vi "TwoBallAuton3-12-14.vi"() -> ()   [LabVIEW 2014]
uses:
  TwoBallAuton.ctl
  Events.vi
  AutonVars.vi
panel:
  out "TargetDistance (In) ToReload":dbl=132.0
  out "Time Target (s)":dbl=3.0
  out "Y-Axis (Backward Speed)":dbl
  out "TargetDistance (In) ToFire":dbl=72.0
  out "Finish?":bool
  out "State":T1=enum."GetBall"
  # "Variables"
  # "Outputs"
  # "Inputs"
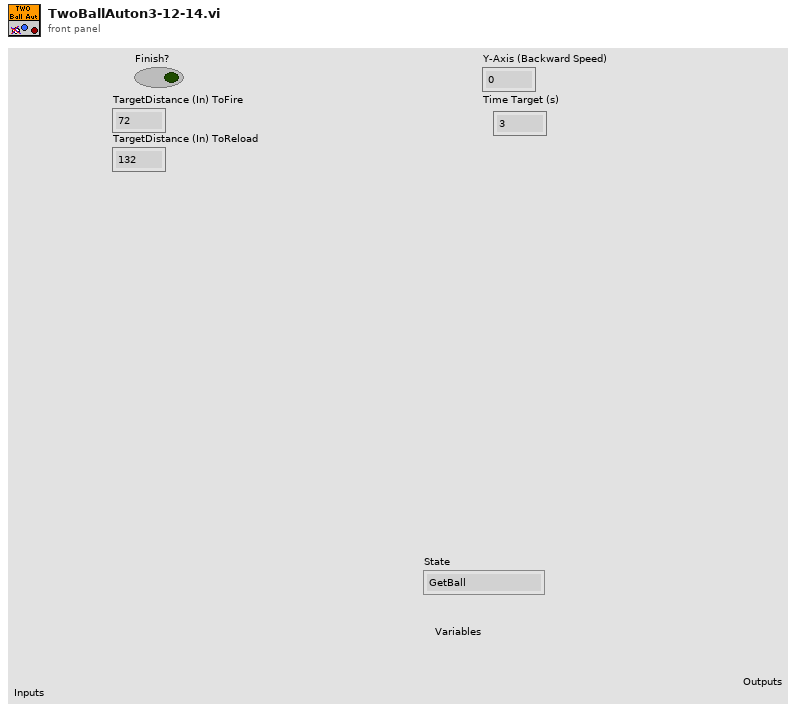
[diagram p1: front panel]
types:
  T1 = typedef "TwoBallAuton.ctl" = enum16{"Start", "LineUp", "Fire", "Reload", "GetBall", "Finish"}
  T2 = cluster{"Translate":dbl, "Y-Axis (Backward Speed)":dbl, "Rotate":dbl, "Tank right side":dbl, "axis 5":dbl, "axis 6":dbl, "Use gyro":bool, "Exponential\ndrive":bool, "Ring light":bool, "PID rotation":bool, "PID Gain":dbl}
  T3 = typedef "Eventgrab.ctl" = cluster{"Grab":bool, "GroundPass":bool, "Test Aqaure":dbl, "Shoulder up or down?":bool, "Auton drag":bool}
  T4 = cluster{"Reloading?":bool, "Throw":bool, "Ready?":bool, "Truss throw":bool, "Power is high?":bool, "Automatic relaod?":bool, "Manuall servo":bool}
  T5 = typedef "WPI_SolenoidValue.ctl" = enum16{"Off", "On", "Forward", "Reverse"}
  T6 = cluster{"Ultrasonic Distance (In)":dbl, "Gyro":dbl, "TopAquisition sensor":bool, "Encoder distance":dbl, "Encoder rate":dbl, "Encoder direction":bool, "winch engaged?":T5, "Motor Values":dbl[], "Latch encoder":u32, "BottomAquistion":bool, "BottomAquistion 2":bool, "Gyro Rate":dbl}
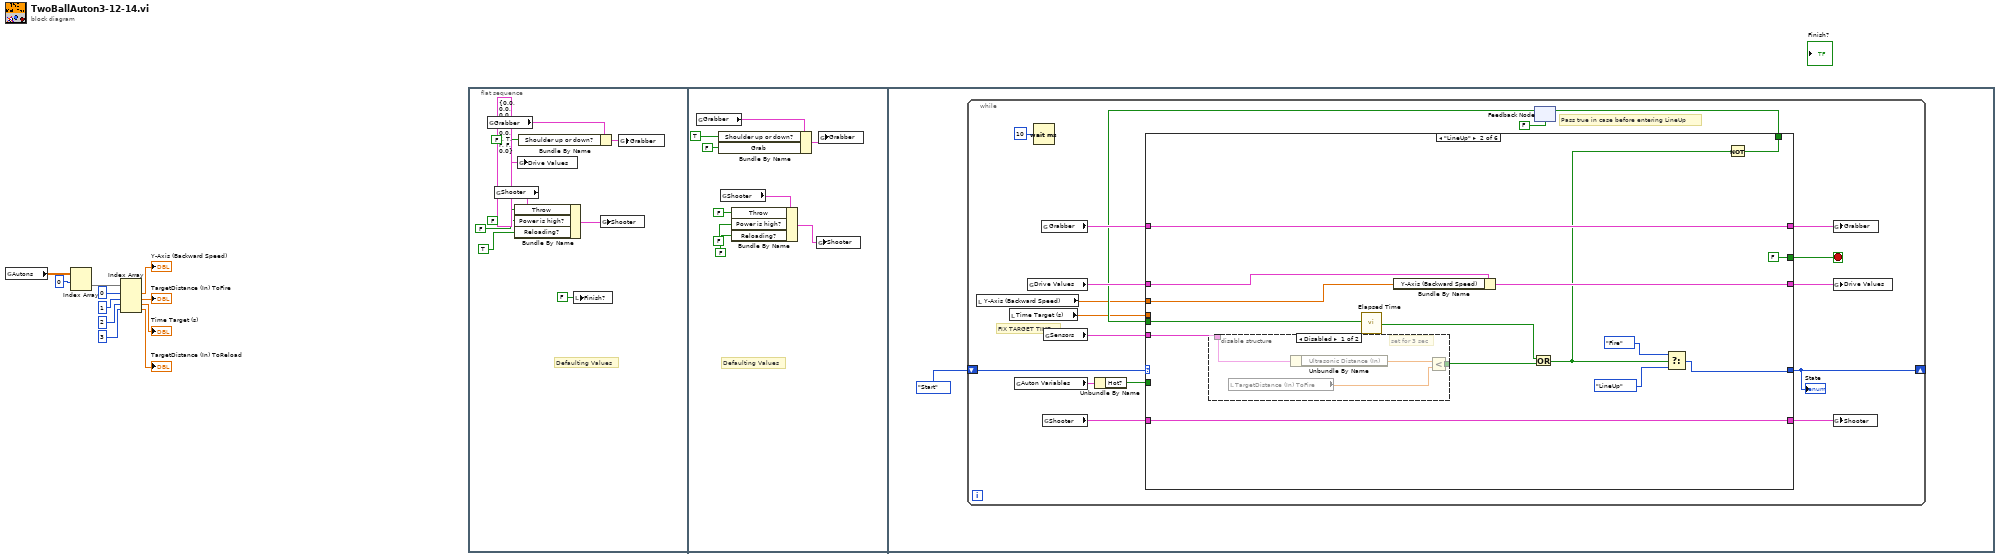
[diagram p0: block diagram]
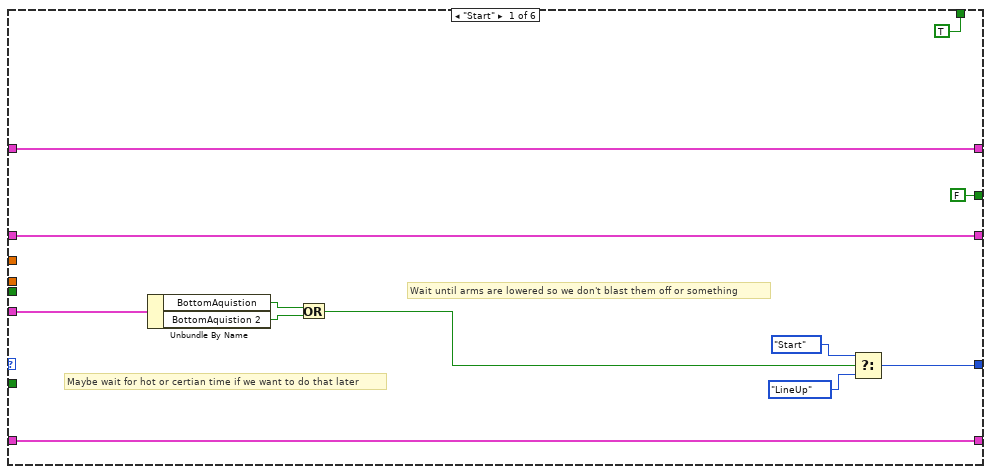
[diagram p2: hidden frame]
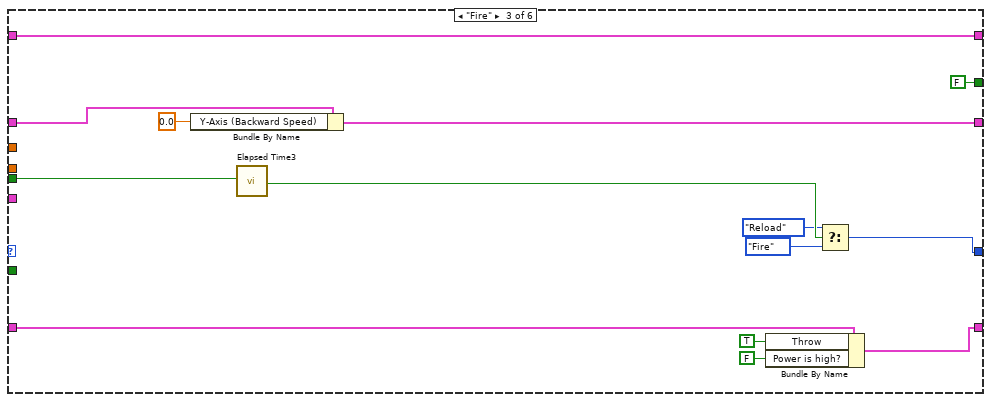
[diagram p4: hidden frame]
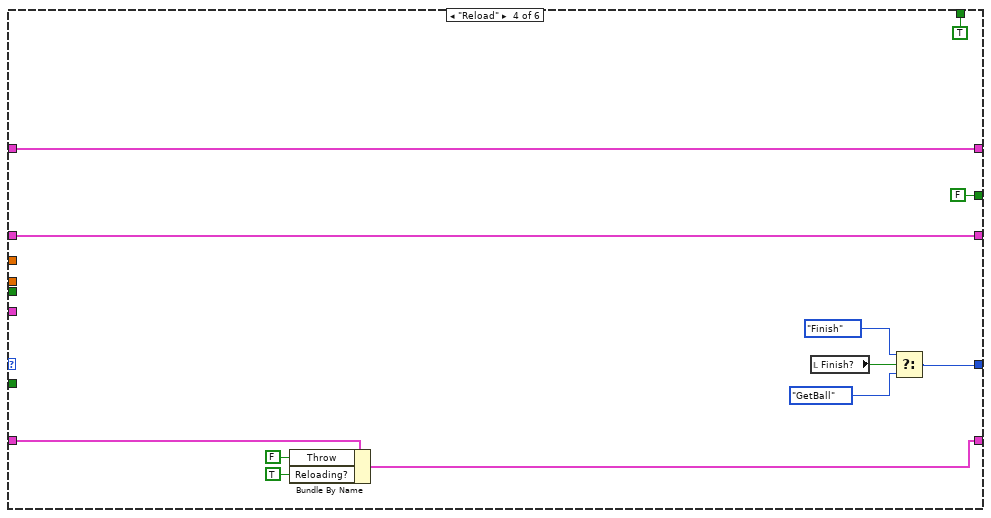
[diagram p5: hidden frame]
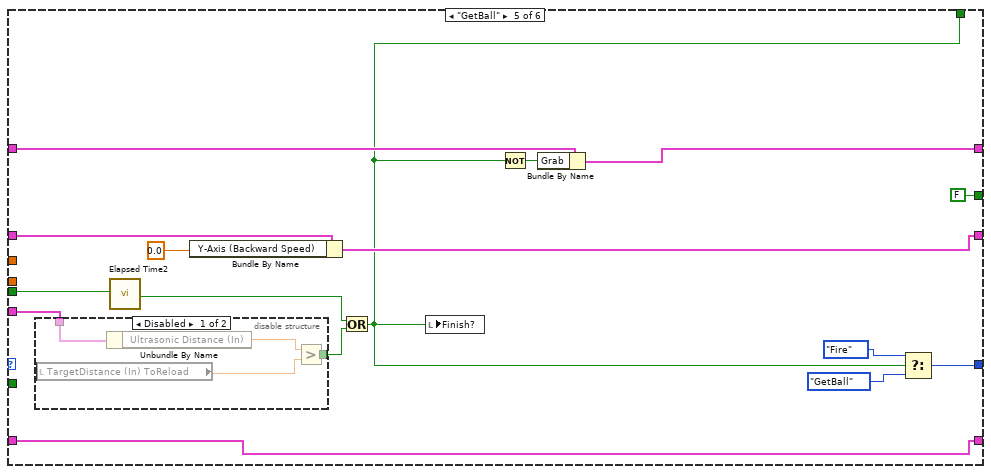
[diagram p6: hidden frame]
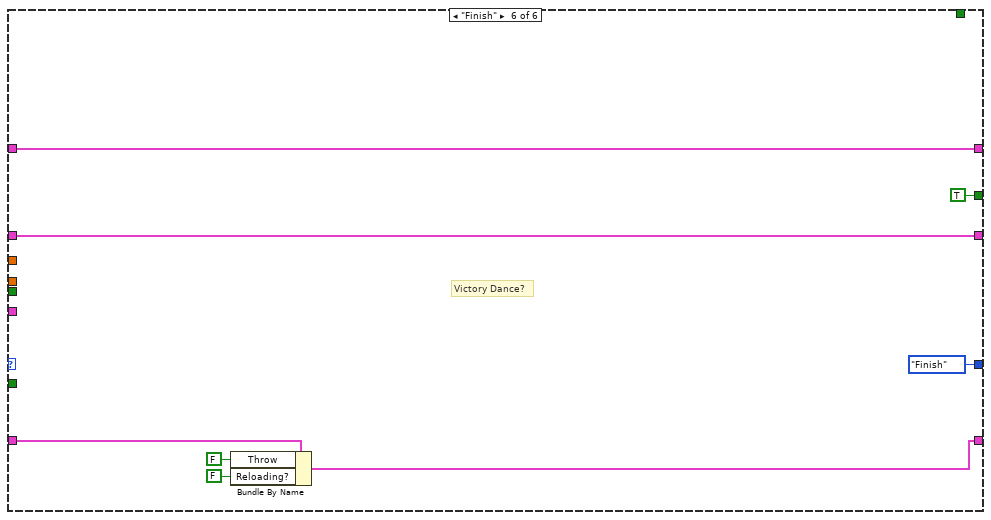
[diagram p8: hidden frame]
diagram:
  n1 = global read "AutonVars.vi" "Autons"() -> (w8:dbl[][])
  n2 = Index Array(array=w8, index (row)=0) -> (element=w6:dbl[])  [unwired: 1 in]
  n3 = Index Array(array=w6, index #1=0 ("index"), index #2=1 ("index"), index #3=2 ("index"), index #4=3 ("index")) -> (element #1=→"Y-Axis (Backward Speed)":dbl, element #2=→"TargetDistance (In) ToFire":dbl, element #3=→"Time Target (s)":dbl, element #4=→"TargetDistance (In) ToReload":dbl)
  n4 = flat-sequence {
    frame #0 {
      # "Defaulting Values"
      n5 = global read "Events.vi" "Grabber"() -> (w20:T3)
      n6 = global read "Events.vi" "Shooter"() -> (w18:T4)
      n7 = Bundle By Name(cluster=w18, "Throw"=FALSE, "Power is high?"=FALSE, "Reloading?"=TRUE) -> (w17:T4)
      n8 = global write "Events.vi" "Drive Values"(T2 {"Translate"=0.0, "Y-Axis (Backward Speed)"=0.0, "Rotate"=0.0, "Tank right side"=0.0, "axis 5"=0.0, "axis 6"=0.0, "Use gyro"=FALSE, "Exponential\ndrive"=TRUE, "Ring light"=FALSE, "PID rotation"=FALSE, "PID Gain"=0.0} ("Drive Values")) -> ()
      n9 = Bundle By Name(cluster=w20, "Shoulder up or down?"=FALSE) -> (w21:T3)
      n10 = local write "Finish?"(FALSE ("Finish?")) -> ()
      n11 = global write "Events.vi" "Shooter"(w17) -> ()
      n12 = global write "Events.vi" "Grabber"(w21) -> ()
    }
    frame #1 {
      # "Defaulting Values"
      n13 = global read "Events.vi" "Grabber"() -> (w24:T3)
      n14 = Bundle By Name(cluster=w24, "Shoulder up or down?"=TRUE, "Grab"=FALSE) -> (w25:T3)
      n15 = global read "Events.vi" "Shooter"() -> (w30:T4)
      n16 = Bundle By Name(cluster=w30, "Throw"=FALSE, "Power is high?"=FALSE, "Reloading?"=FALSE) -> (w29:T4)
      n17 = global write "Events.vi" "Shooter"(w29) -> ()
      n18 = global write "Events.vi" "Grabber"(w25) -> ()
    }
    frame #2 {
      n19 = while {
        shift-right: [w42] -> _
        shift-left: TwoBallAuton."Start" -> [w43]
        stop <- w37 stop-if-true
        # "FIX TARGET TIME"
        # "Pass true in case before entering LineUp"
        n20 = local read "Y-Axis (Backward Speed)"() -> (w32:dbl)
        n21 = local read "Time Target (s)"() -> (w33:dbl)
        n22 = global read "Events.vi" "Auton Variables"() -> (w45:cluster{"Hot?":bool, "WhichAuton":string})
        n23 = global read "Events.vi" "Drive Values"() -> (w47:T2)
        n24 = Wait (ms)(milliseconds to wait=u32 10) -> ()  [unwired: 1 out]
        n25 = global read "Events.vi" "Grabber"() -> (w46:T3)
        n26 = global read "Events.vi" "Shooter"() -> (w48:T4)
        n27 = global read "Events.vi" "Sensors"() -> (w38:T6)
        n28 = Unbundle By Name(w45) -> ("Hot?"=w44:bool)
        n29 = feedback #1(FALSE) -> (w35:bool)
        n30 = case shown="\"LineUp\"" w43 {
          tunnel: w44 -> [_ _ _ _ _ _]
          tunnel: w48 -> [w59 w75 w87 w105 w108 w128]
          tunnel: w47 -> [w60 w67 w93 w96 w116 w133]
          tunnel: w46 -> [w61 w76 w90 w97 w122 w134]
          tunnel: [w51 w71 w84 w101 w112 TwoBallAuton."Finish" ("f")] -> w42
          tunnel: [w61 w76 w90 w97 w110 w134] -> w41
          tunnel: [w60 w73 w92 w96 w115 w133] -> w40
          tunnel: [w59 w75 w86 w102 w108 w127] -> w39
          tunnel: w38 -> [w57 w66 _ _ w120 _]
          tunnel: [FALSE FALSE FALSE FALSE FALSE TRUE] -> w37
          tunnel: w35 -> [_ w65 w85 _ w121 _]
          tunnel: [TRUE w63 _ TRUE w111 _] -> w36
          tunnel: w33 -> [_ _ _ _ _ _]
          tunnel: w32 -> [_ w64 _ _ _ _]
          frame "Start" {
            # "Wait until arms are lowered so we don't blast them off or something"
            # "Maybe wait for hot or certian time if we want to do that later"
            n31 = Unbundle By Name(w57) -> ("BottomAquistion"=w55:bool, "BottomAquistion 2"=w56:bool)
            n32 = Or(x=w55, y=w56) -> (x .or. y?=w52:bool)
            n33 = Select(t=TwoBallAuton."Start", s=w52, f=TwoBallAuton."LineUp") -> (s? t:f=w51:T1)
          }
          frame "LineUp" {
            n34 = disable-structure shown="Disabled" {
              disable-tunnel: [w79 _] -> w68
              disable-tunnel: w66 -> [w78 _]
              frame Disabled {
                # "set for 3 sec"
                n35 = local read "TargetDistance (In) ToFire"() -> (w77:dbl)
                n36 = Unbundle By Name(w78) -> ("Ultrasonic Distance (In)"=w80:dbl)
                n37 = Less?(x=w80, y=w77) -> (x < y?=w79:bool)
              }
              frame Enabled {
              }
            }
            n38 = call "Elapsed Time"("Reset"=w65) -> ("Time has Elapsed"=w69:bool)  [unwired: 11 in, 7 out]
            n39 = Bundle By Name(cluster=w67, "Y-Axis (Backward Speed)"=w64) -> (w73:T2)
            n40 = Or(x=w69, y=w68) -> (x .or. y?=w62:bool)
            n41 = Select(t=TwoBallAuton."Fire", s=w62, f=TwoBallAuton."LineUp") -> (s? t:f=w71:T1)
            n42 = Not(x=w62) -> (.not. x?=w63:bool)
          }
          frame "Fire" {
            n43 = Bundle By Name(cluster=w93, "Y-Axis (Backward Speed)"=0.0 ("Forward Speed")) -> (w92:T2)
            n44 = call "Elapsed Time3"("Reset"=w85) -> ("Time has Elapsed"=w82:bool)  [unwired: 11 in, 7 out]
            n45 = Bundle By Name(cluster=w87, "Throw"=TRUE, "Power is high?"=FALSE) -> (w86:T4)
            n46 = Select(t=TwoBallAuton."Reload", s=w82, f=TwoBallAuton."Fire") -> (s? t:f=w84:T1)
          }
          frame "Reload" {
            n47 = Bundle By Name(cluster=w105, "Throw"=FALSE, "Reloading?"=TRUE) -> (w102:T4)
            n48 = local read "Finish?"() -> (w100:bool)
            n49 = Select(t=TwoBallAuton."Finish", s=w100, f=TwoBallAuton."GetBall") -> (s? t:f=w101:T1)
          }
          frame "GetBall" {
            n50 = disable-structure shown="Disabled" {
              disable-tunnel: w120 -> [w126 _]
              disable-tunnel: [w124 _] -> w119
              frame Disabled {
                n51 = local read "TargetDistance (In) ToReload"() -> (w123:dbl)
                n52 = Unbundle By Name(w126) -> ("Ultrasonic Distance (In)"=w125:dbl)
                n53 = Greater?(x=w125, y=w123) -> (0:w124:bool)
              }
              frame Enabled {
              }
            }
            n54 = call "Elapsed Time2"("Reset"=w121) -> ("Time has Elapsed"=w118:bool)  [unwired: 11 in, 7 out]
            n55 = Bundle By Name(cluster=w116, "Y-Axis (Backward Speed)"=0.0) -> (w115:T2)
            n56 = Or(x=w118, y=w119) -> (x .or. y?=w111:bool)
            n57 = local write "Finish?"(w111) -> ()
            n58 = Not(x=w111) -> (.not. x?=w117:bool)
            n59 = Bundle By Name(cluster=w122, "Grab"=w117) -> (w110:T3)
            n60 = Select(t=TwoBallAuton."Fire", s=w111, f=TwoBallAuton."GetBall") -> (s? t:f=w112:T1)
          }
          frame "Finish" {
            # "Victory Dance?"
            n61 = Bundle By Name(cluster=w128, "Throw"=FALSE, "Reloading?"=FALSE) -> (w127:T4)
          }
        }
        "State" <- w42
        n62 = feedback-in #1(w36) -> ()
        n63 = global write "Events.vi" "Grabber"(w41) -> ()
        n64 = global write "Events.vi" "Drive Values"(w40) -> ()
        n65 = global write "Events.vi" "Shooter"(w39) -> ()
      }
    }
  }
